vi "Get Acquisition Progress.vi"(8 "error in (no error)":errorcluster, 10 "series":i32, 11 "acc":i32) -> (0 "error out":errorcluster, 1 "function return":u32, 2 "series out":i32, 3 "acc out":i32)   [LabVIEW 2014, in "atmcd32d.lvlib"]
doc: "unsigned int WINAPI GetAcquisitionProgress(long * acc, long * series);"
uses:
  atmcd32d.lvlib
  atmcd32d.dll
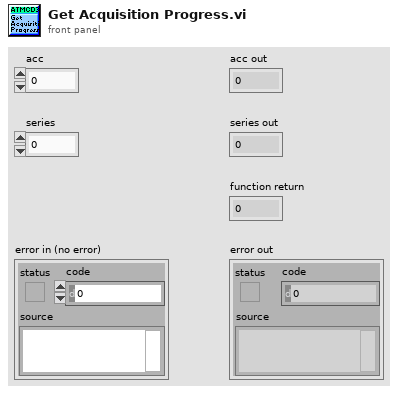
[diagram p1: front panel]
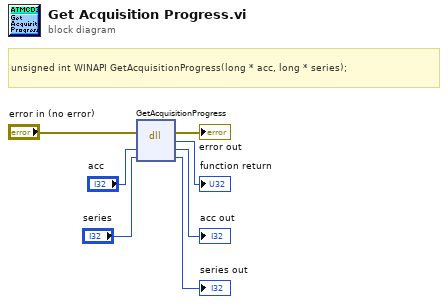
[diagram p0: block diagram]
diagram:
  # "unsigned int WINAPI GetAcquisitionProgress(long * acc, long * series);"
  n1 = dll-call lib="C:/Users/Bakir/Documents/Lambda2-Testing/lib/Andorlib/atmcd32d.*" fn="GetAcquisitionProgress"(error in="error in (no error)", "acc"="acc", "series"="series") -> (error out=→"error out":errorcluster, →"function return":u32, "acc"=→"acc out":i32, "series"=→"series out":i32)  [unwired: 2 in, 1 out]
